vi "Query USIM XOR Res Length.vi"(8 "error in (no error)":errorcluster, 10 "SIM Profile (\"SIM1\")":string="SIM1", 11 "VISA resource name":refnum<visa-resource-name>) -> (0 "error out":errorcluster, 2 "Length":i32, 3 "VISA resource name out":refnum<visa-resource-name>)   [LabVIEW 2015, in "Rohde&Schwarz CMXP Base.lvlib"]
doc: "Queries the length of the RES (L2) for XOR authentication algorithms.\n\nAttribute:\n-\n\nRemote-control command:\n[CONFigure:]SIMProfile:USIM:SECurity:XORLength?"
uses:
  <instrlib>/Rohde&Schwarz CMXP Base/Rohde&Schwarz CMXP Base.lvlib
  <instrlib>/Rohde&Schwarz CMXP Base/Private/rsidr_core.llb/rsidr_core.lvlib
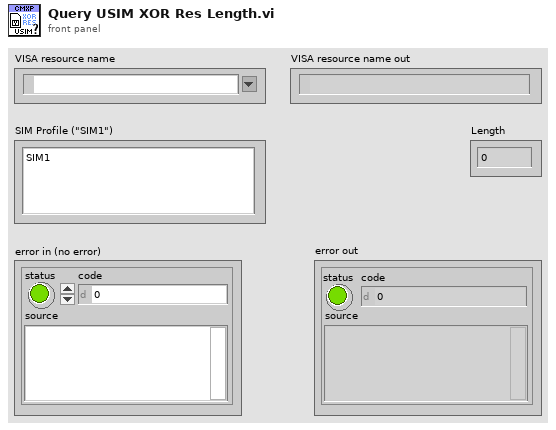
[diagram p1: front panel]
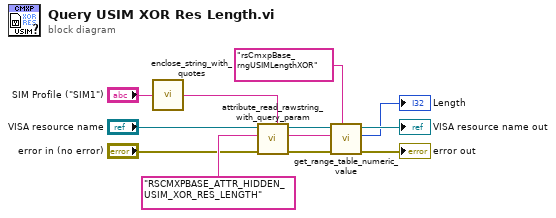
[diagram p0: block diagram]
diagram:
  n1 = call <instrlib>:"enclose_string_with_quotes.vi"("String to enclose"="SIM Profile (\"SIM1\")") -> ("String out"=w1:string)  [unwired: 4 in]
  n2 = call <instrlib>:"attribute_read_rawstring_with_query_param.vi"("Query Parameter (None)"=w1, "error in"="error in (no error)", "Attribute ID"="RSCMXPBASE_ATTR_HIDDEN_USIM_XOR_RES_LENGTH", "VISA resource name"="VISA resource name") -> ("error out"=w10:errorcluster, "RawString out"=w9:string, "VISA resource name out"=w11:refnum<visa-resource-name>)  [unwired: 5 in]
  n3 = call <instrlib>:"get_range_table_numeric_value.vi"("Range Table ID in"="rsCmxpBase_rngUSIMLengthXOR", "error in"=w10, "String Value"=w9, "VISA resource name"=w11) -> ("error out"=→"error out":errorcluster, "I32 output"=→"Length":i32, "VISA resource name out"=→"VISA resource name out":refnum<visa-resource-name>)  [unwired: 5 in]
